vi "ICP_preALIGNMENT_LV2010.vi"(0 "X_target":sgl[][](array[numeric])=[[1.05222, 0.302594, -0.0318983, -0.0347655, 0.2393]], 1 "Y_target":sgl[][](array[numeric])=[[-0.151883, -0.473106, 0.667105, 0.854581, -0.277468]], 3 "icp_maxCorrespondence_distance":dbl=1.0, 4 "icp_Transformation_epsilon:1E-8":dbl=1e-08, 5 "Z_target":sgl[][](array[numeric])=[[-0.106395, 0.292602, 0.441304, -0.0361733, -0.916762]], 7 "X_source":sgl[][](array[numeric])=[[0.352222, -0.397406, -0.731898, -0.734766, -0.4607]], 8 "icp_RANSAC_threshold:0.05":dbl=0.05, 9 "Y_source":sgl[][](array[numeric])=[[-0.151883, -0.473106, 0.667105, 0.854581, -0.277468]], 10 "full_registration (0 full, < 0 icp only, > 0 sac-ia only)":i32, 11 "sac_ia_maximum_iterations":i32, 12 "sac_ia_max_correspondence_distance":sgl, 13 "icp_EuclideanFitness_epsilon":dbl=1.0, 14 "sac_ia_min_sample_distance":sgl, 16 "icp_maxICP_iterations:15":i32=20, 17 "Z_source":sgl[][](array[numeric])=[[-0.106395, 0.292602, 0.441304, -0.0361733, -0.916762]], 18 "normals_radius":dbl format="%#_13g", 19 "fpfh_radius":dbl format="%#_13g") -> (20 "transformation_matrix":sgl[][](array[numeric])=[[1.0000002, 2.1462839e-07, -1.6423296e-07, 0.7000001], [-1.3767561e-07, 1.0, -6.5921284e-08, -7.4505806e-08], [1.6773438e-07, 2.9214991e-08, 1.0, 9.313226e-08], [0.0, 0.0, 0.0, 1.0]], 21 "score":dbl=1.0883044465614945e-12, 22 "icprot":sgl[][](array[numeric]), 23 "rotation angles [rad]":T1={"Rx angle [rad]"=2.9214991e-08, "Ry angle [rad]"=-1.6773438e-07, "Rz angle [rad]"=-1.3767558e-07}, 24 "processing time [ms]":u32=43, 25 "converged?":bool=TRUE, 26 "OUT":dbl[][](array[numeric]), 27 "UPDATE?":bool)   [LabVIEW 2012]
uses:
  <vilib>/Analysis/baseanly.llb/Real A x B.vi
  <vilib>/Analysis/Matrix/Numeric/Conversions/Matrix To Array - RM.vi
  <vilib>/Analysis/Matrix/Numeric/Conversions/Array To Matrix - RA2.vi
  ICP_PCL_preALIGNMENT.dll
  <vilib>/Analysis/NI_AALBase.lvlib
  <vilib>/Analysis/Matrix/NI_Matrix.lvlib
panel:
  out "sqrt(x)":dbl[](array[numeric])
  out "XY Graph":cluster{"Y":dbl[], "Y":dbl[]}[](graph)
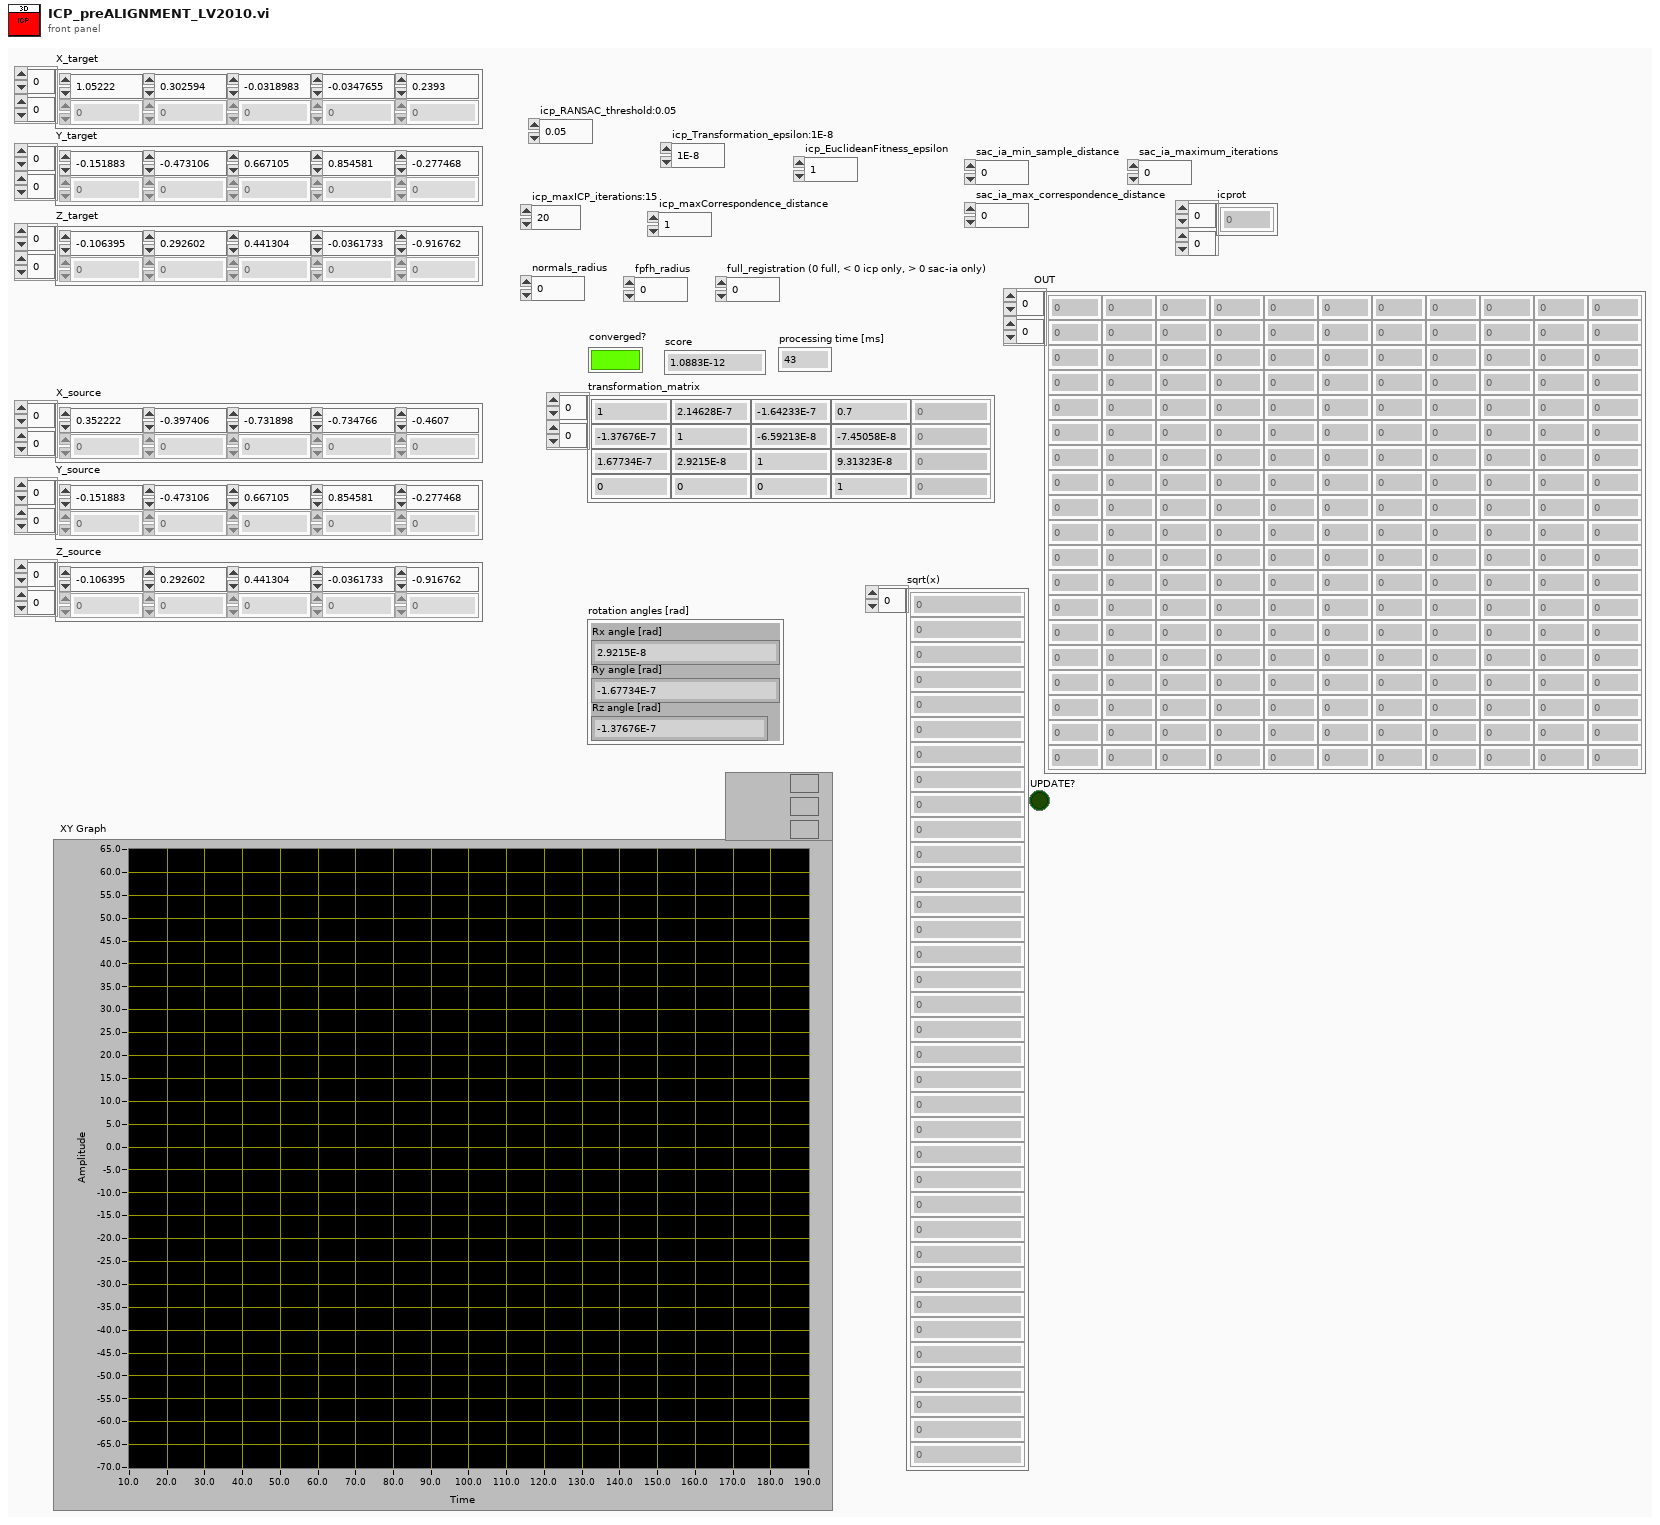
[diagram p1: front panel]
types:
  T1 = cluster{"Rx angle [rad]":sgl, "Ry angle [rad]":sgl, "Rz angle [rad]":sgl}
  T2 = typedef "NI_Matrix.lvlib/RealMatrix.ctl" = dbl[][]
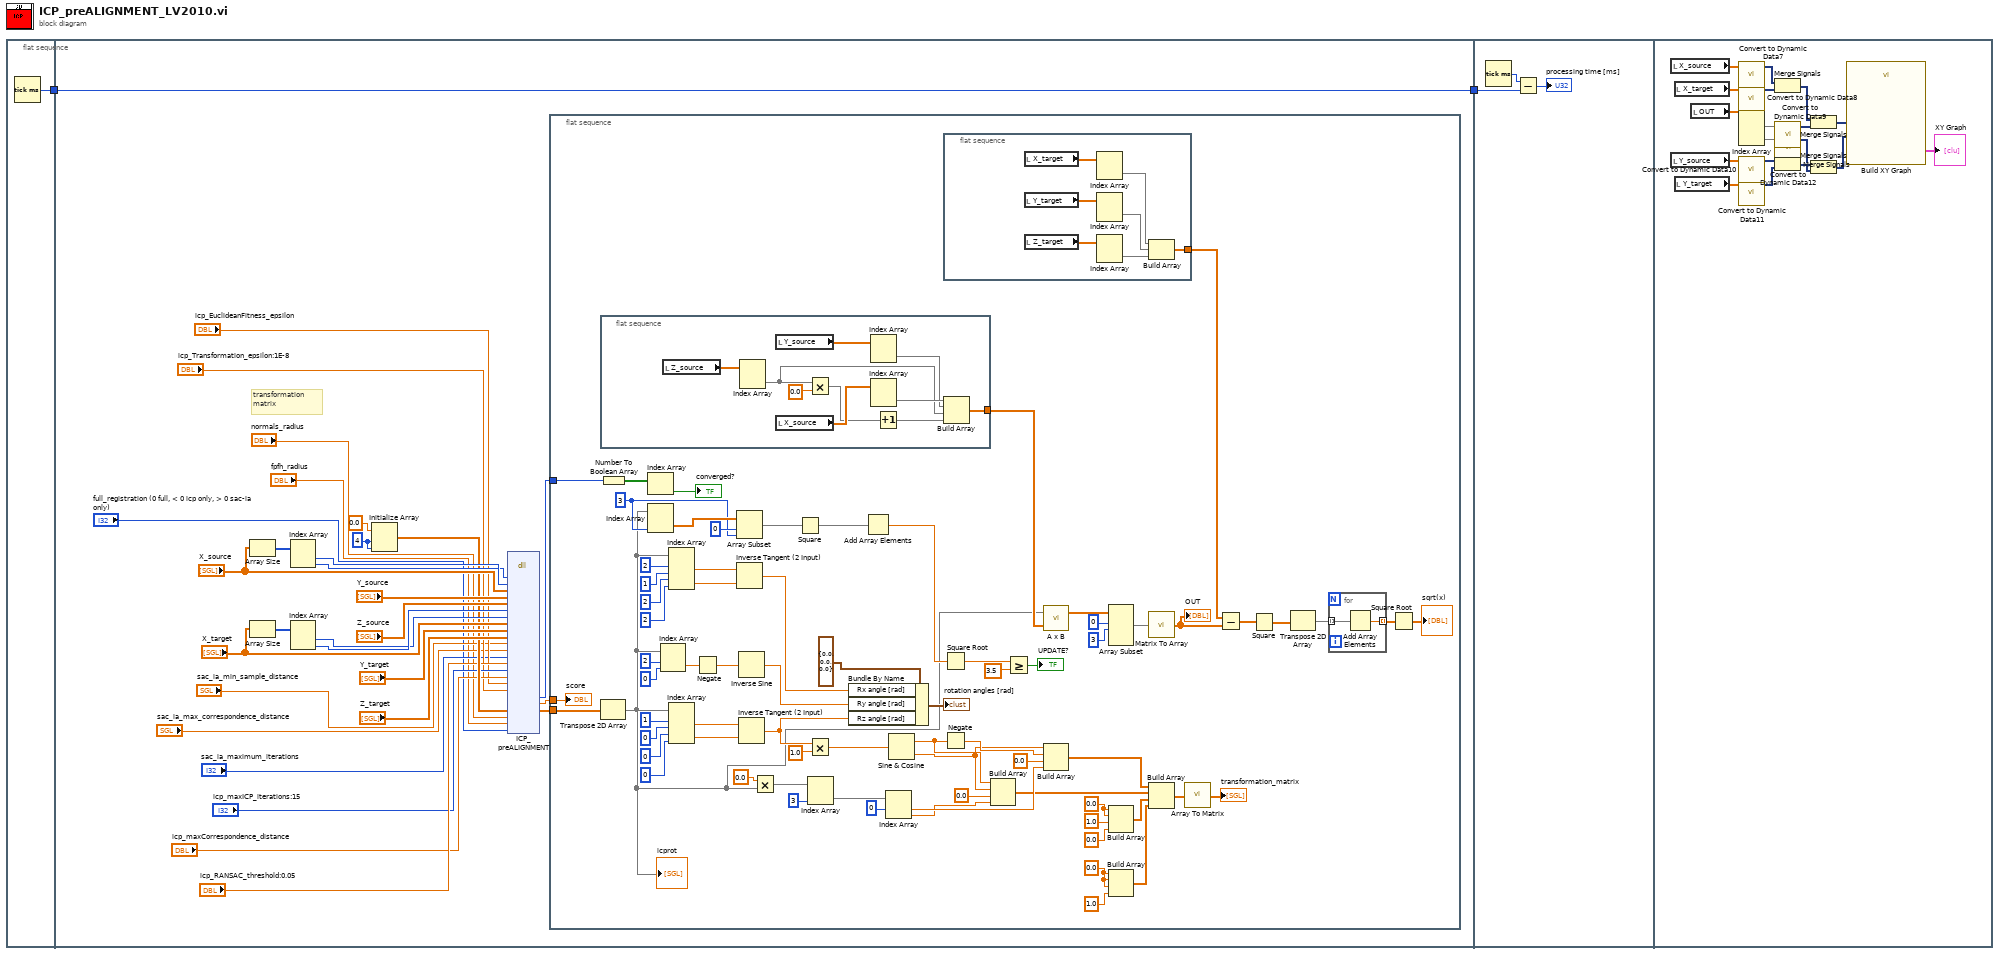
[diagram p0: block diagram]
diagram:
  n1 = flat-sequence {
    tunnel: [w3] -> w1
    tunnel: [w4] -> w2
    tunnel: w1 -> [w4]
    tunnel: w2 -> [w126]
    frame #0 {
      n2 = Tick Count (ms)() -> (millisecond timer value=w3:u32)
    }
    frame #1 {
      w8 = 4 ("dimension size")
      # "transformation \nmatrix"
      n3 = Array Size(array="X_source") -> (size(s)=w6:i32[])
      n4 = Array Size(array="X_target") -> (size(s)=w5:i32[])
      n5 = Index Array(array=w6) -> (element #1=w30:i32, element #2=w29:i32)  [unwired: 2 in]
      n6 = Index Array(array=w5) -> (element #1=w24:i32, element #2=w25:i32)  [unwired: 2 in]
      n7 = Initialize Array(sgl 0.0 ("element"), w8, w8) -> (w23:sgl[][])
      n8 = dll-call lib="C:/eurecar/3d/ICP_PCL_preALIGNMENT.dll" fn="ICP_preALIGNMENT"("cloudCols_source"=w29, "cloudRows_source"=w30, "cloudX_source"="X_source", "cloudY_source"="Y_source", "cloudZ_source"="Z_source", "cloudCols_target"=w25, "cloudRows_target"=w24, "cloudX_target"="X_target", "cloudY_target"="Y_target", "cloudZ_target"="Z_target", "sac_ia_min_sample_distance"="sac_ia_min_sample_distance", "sac_ia_max_correspondence_distance"="sac_ia_max_correspondence_distance", "sac_ia_maximum_iterations"="sac_ia_maximum_iterations", "icp_RANSAC_threshold"="icp_RANSAC_threshold:0.05", "icp_maxICP_iterations"="icp_maxICP_iterations:15", "icp_maxCorrespondence_distance"="icp_maxCorrespondence_distance", "icp_EuclideanFitness_epsilon"="icp_EuclideanFitness_epsilon", "icp_Transformation_epsilon"="icp_Transformation_epsilon:1E-8", "final_transformation_matrix"=w23, "normals_radius"="normals_radius", "fpfh_radius"="fpfh_radius", "full_registration"="full_registration (0 full, < 0 icp only, > 0 sac-ia only)") -> ("icp_converged"=w11:i32, "icp_score"=w10:dbl, "final_transformation_matrix"=w7:sgl[][])  [unwired: 27 in, 2 out]
      n9 = flat-sequence {
        tunnel: w11 -> [w105]
        tunnel: w10 -> [w103]
        tunnel: w7 -> [w102]
        frame #0 {
          w35 = 0.0 ("element")
          w45 = 0.0 ("element")
          w67 = 3 ("disabled index (col)")
          n10 = flat-sequence {
            tunnel: [w116] -> w81
            frame #0 {
              n11 = local read "Z_source"() -> (w123:sgl[][])
              n12 = Index Array(array=w123) -> (element=w120:sgl[])  [unwired: 2 in]
              n13 = local read "Y_source"() -> (w124:sgl[][])
              n14 = local read "X_source"() -> (w125:sgl[][])
              n15 = Multiply(x=w120, y=sgl 0.0) -> (x*y=w118:sgl[])
              n16 = Index Array(array=w124) -> (element=w121:sgl[])  [unwired: 2 in]
              n17 = Index Array(array=w125) -> (element=w122:sgl[])  [unwired: 2 in]
              n18 = Increment(x=w118) -> (x+1=w117:sgl[])
              n19 = Build Array(w122, w121, w120, w117) -> (w116:sgl[][])
            }
          }
          n20 = Transpose 2D Array(2D array=w102) -> (transposed array=w57:sgl[][])
          "icprot" <- w57
          n21 = Number To Boolean Array(number=w105) -> (Boolean array=w106:bool[])
          n22 = Index Array(array=w106) -> (element=→"converged?":bool)  [unwired: 1 in]
          n23 = Index Array(array=w57, index (col)=w67) -> (element=w69:sgl[])  [unwired: 1 in]
          n24 = Index Array(array=w57, index (row)=2, index (col)=0 ("disabled index (col)")) -> (element=w99:sgl)
          n25 = Index Array(array=w57, index (row) #1=2 ("index (row)"), index (col) #1=1 ("disabled index (col)"), index (row) #2=2 ("index (row)"), index (col) #2=2 ("index (row)")) -> (element #1=w93:sgl, element #2=w92:sgl)
          n26 = Index Array(array=w57, index (row) #1=1 ("index (row)"), index (col) #1=0 ("disabled index (col)"), index (row) #2=0 ("index (row)"), index (col) #2=0 ("index (row)")) -> (element #1=w90:sgl, element #2=w91:sgl)
          n27 = Negate(x=w99) -> (-x=w98:sgl)
          n28 = Array Subset(array=w69, index=0, length=w67) -> (w66:sgl[])
          n29 = Inverse Tangent (2 Input)(1:w92, 2:w93) -> (0:w84:sgl)
          n30 = Inverse Sine(1:w98) -> (0:w83:sgl)
          n31 = Inverse Tangent (2 Input)(1:w91, 2:w90) -> (0:w60:sgl)
          n32 = Multiply(x=sgl 0.0 ("y"), y=w57) -> (x*y=w56:sgl[][])
          n33 = Square(x=w66) -> (x^2=w65:sgl[])
          n34 = Multiply(x=w60, y=sgl 1.0) -> (x*y=w59:sgl)
          n35 = Index Array(array=w56, index (col)=3 ("disabled index (col)")) -> (element=w54:sgl[])  [unwired: 1 in]
          n36 = Bundle By Name(cluster=T1 {"Rx angle [rad]"=0.0, "Ry angle [rad]"=0.0, "Rz angle [rad]"=0.0} ("input cluster"), "Rx angle [rad]"=w84, "Ry angle [rad]"=w83, "Rz angle [rad]"=w60) -> (→"rotation angles [rad]":T1)
          n37 = Add Array Elements(numeric array=w65) -> (sum=w64:sgl)
          n38 = Index Array(array=w54, index #1=0 ("index")) -> (element #1=w50:sgl, element #2=w46:sgl)  [unwired: 1 in]
          n39 = Sine & Cosine(0:w59) -> (1:w49:sgl, 2:w48:sgl)
          n40 = Square Root(x=w64) -> (sqrt(x)=w63:sgl)
          n41 = Negate(x=w49) -> (-x=w52:sgl)
          n42 = flat-sequence {
            tunnel: [w109] -> w75
            frame #0 {
              n43 = local read "X_target"() -> (w115:sgl[][])
              n44 = local read "Y_target"() -> (w114:sgl[][])
              n45 = local read "Z_target"() -> (w113:sgl[][])
              n46 = Index Array(array=w115) -> (element=w112:sgl[])  [unwired: 2 in]
              n47 = Index Array(array=w114) -> (element=w111:sgl[])  [unwired: 2 in]
              n48 = Index Array(array=w113) -> (element=w110:sgl[])  [unwired: 2 in]
              n49 = Build Array(w112, w111, w110) -> (w109:sgl[][])
            }
          }
          n50 = Build Array(w49, w48, sgl 0.0 ("element"), w46) -> (w40:sgl[])
          n51 = Greater Or Equal?(x=w63, y=sgl 3.5) -> (x >= y?=→"UPDATE?":bool)
          n52 = call-poly <vilib>:"A x B.vi"("B"=w81, "A"=w57) -> ("A x B"=w80:T2)  [unwired: 1 out]
          n53 = Build Array(w48, w52, sgl 0.0 ("element"), w50) -> (w41:sgl[])
          n54 = Array Subset(array=w80, index (row)=0 ("index"), length (row)=3 ("length")) -> (w77:T2)  [unwired: 2 in]
          n55 = Build Array(w45, w45, 1.0 ("element"), 0.0 ("element")) -> (w39:dbl[])
          n56 = Build Array(w35, w35, w35, 1.0 ("element")) -> (w38:dbl[])
          n57 = call-poly <vilib>:"Matrix To Array.vi"("Real Matrix"=w77) -> ("Real 2D Array"=w76:dbl[][])
          "OUT" <- w76
          n58 = Build Array(w41, w40, w39, w38) -> (w37:dbl[][])
          n59 = call-poly <vilib>:"Array To Matrix.vi"("Real 2D Array"=w37) -> ("Real Matrix"=→"transformation_matrix":T2)
          n60 = Subtract(x=w75, y=w76) -> (x-y=w74:dbl[][])
          n61 = Square(x=w74) -> (x^2=w73:dbl[][])
          n62 = Transpose 2D Array(2D array=w73) -> (transposed array=w72:dbl[][])
          n63 = for {
            tunnel: w72 -> [w108] mode=indexing
            tunnel: [w107] -> w71 mode=indexing
            n64 = Add Array Elements(numeric array=w108) -> (sum=w107:dbl)
          }
          n65 = Square Root(x=w71) -> (sqrt(x)=→"sqrt(x)":dbl[])
          "score" <- w103
        }
      }
    }
    frame #2 {
      n66 = Tick Count (ms)() -> (millisecond timer value=w128:u32)
      n67 = Subtract(x=w128, y=w126) -> (x-y=→"processing time [ms]":u32)
    }
    frame #3 {
      n68 = local read "X_source"() -> (w144:sgl[][])
      n69 = local read "Y_source"() -> (w136:sgl[][])
      n70 = local read "X_target"() -> (w141:sgl[][])
      n71 = local read "Y_target"() -> (w133:sgl[][])
      n72 = local read "OUT"() -> (w145:dbl[][])
      n73 = call "Convert to Dynamic Data7"("2D Array"=w144) -> ("Dynamic Data Type"=w143:dynamicdata)  [unwired: 3 in]
      n74 = call "Convert to Dynamic Data8"("2D Array"=w141) -> ("Dynamic Data Type"=w140:dynamicdata)  [unwired: 3 in]
      n75 = Index Array(array=w145) -> (element #1=w138:dbl[], element #2=w130:dbl[])  [unwired: 4 in]
      n76 = call "Convert to Dynamic Data10"("2D Array"=w136) -> ("Dynamic Data Type"=w135:dynamicdata)  [unwired: 3 in]
      n77 = call "Convert to Dynamic Data11"("2D Array"=w133) -> ("Dynamic Data Type"=w132:dynamicdata)  [unwired: 3 in]
      n78 = Merge Signals(w143, w140) -> (w142:dynamicdata)
      n79 = call "Convert to Dynamic Data9"("Array"=w138) -> ("Dynamic Data Type"=w137:dynamicdata)  [unwired: 3 in]
      n80 = call "Convert to Dynamic Data12"("Array"=w130) -> ("Dynamic Data Type"=w129:dynamicdata)  [unwired: 3 in]
      n81 = Merge Signals(w135, w132) -> (w134:dynamicdata)
      n82 = Merge Signals(w142, w137) -> (w139:dynamicdata)
      n83 = Merge Signals(w134, w129) -> (w131:dynamicdata)
      n84 = call "Build XY Graph"("Y Input"=w131, "X Input"=w139) -> ("XY Graph"=→"XY Graph":cluster{"Y":dbl[], "Y":dbl[]}[])  [unwired: 3 in, 6 out]
    }
  }
